vi "DriveStateController.vi"   [LabVIEW 2018]
uses:
  instructions.vi
  constants.vi
  outputs.vi
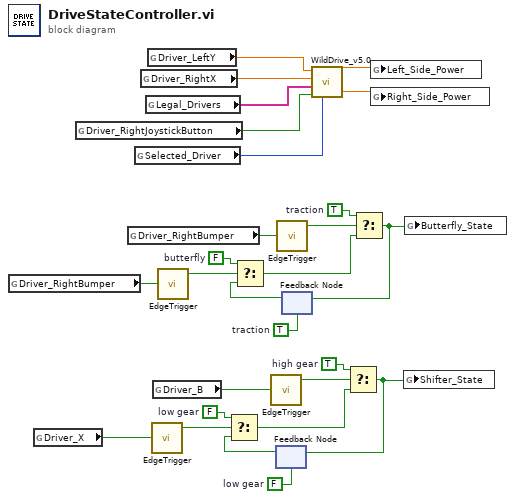
[diagram p0: block diagram]
diagram:
  w2 = FALSE  # low gear
  w5 = TRUE  # high gear
  w8 = FALSE  # low gear
  w12 = TRUE  # traction
  w15 = TRUE  # traction
  w18 = FALSE  # butterfly
  n1 = global read "instructions.vi" "Driver_RightBumper"() -> (w20:bool)
  n2 = global read "instructions.vi" "Driver_X"() -> (w10:bool)
  n3 = global read "instructions.vi" "Driver_RightJoystickButton"() -> (w25:bool)
  n4 = global read "instructions.vi" "Driver_RightBumper"() -> (w17:bool)
  n5 = global read "instructions.vi" "Selected_Driver"() -> (w27:i32)
  n6 = global read "instructions.vi" "Driver_RightX"() -> (w23:dbl)
  n7 = global read "constants.vi" "Legal_Drivers"() -> (w26:string[])
  n8 = global read "instructions.vi" "Driver_LeftY"() -> (w24:dbl)
  n9 = call "EdgeTrigger.vi"("Input Signal"=w10) -> ("Rising Edge Trigger"=w9:bool)  [unwired: 2 out]
  n10 = global read "instructions.vi" "Driver_B"() -> (w7:bool)
  n11 = call "EdgeTrigger.vi"("Input Signal"=w20) -> ("Rising Edge Trigger"=w19:bool)  [unwired: 2 out]
  n12 = call "EdgeTrigger.vi"("Input Signal"=w7) -> ("Rising Edge Trigger"=w6:bool)  [unwired: 2 out]
  n13 = feedback #1(w2) -> (w3:bool)
  n14 = Select(t=w8, s=w9, f=w3) -> (s? t:f=w4:bool)
  n15 = call "EdgeTrigger.vi"("Input Signal"=w17) -> ("Rising Edge Trigger"=w16:bool)  [unwired: 2 out]
  n16 = feedback #2(w12) -> (w13:bool)
  n17 = Select(t=w18, s=w19, f=w13) -> (s? t:f=w14:bool)
  n18 = call "WildDrive_v5.0.vi"("Selected_Driver"=w27, "Super Turn"=w25, "Legal_Drivers"=w26, "Turn Joystick"=w23, "Speed Joystick"=w24) -> ("Right Side Power"=w22:dbl, "Left Side Power"=w21:dbl)  [unwired: 5 in]
  n19 = Select(t=w5, s=w6, f=w4) -> (s? t:f=w1:bool)
  n20 = feedback-in #1(w1) -> ()
  n21 = Select(t=w15, s=w16, f=w14) -> (s? t:f=w11:bool)
  n22 = feedback-in #2(w11) -> ()
  n23 = global write "outputs.vi" "Left_Side_Power"(w21) -> ()
  n24 = global write "outputs.vi" "Right_Side_Power"(w22) -> ()
  n25 = global write "outputs.vi" "Shifter_State"(w1) -> ()
  n26 = global write "outputs.vi" "Butterfly_State"(w11) -> ()
